vi "Stanford Research PS300 Series Configuration Display.vi"() -> ()   [LabVIEW 2013]
doc: "This VI first configures the instrument's setting (voltage/current) plus an associated value, commands the instrument to output the voltage, and finally returns a reading, showing the current display of the output source.\n\nNote: If Err 7 is generated by this VI Check to make sure that the High Vlotage Switch on the Instrument's Front Panel is turned ON, if it is OFF the high voltage will remain off and the instrument generates an execution error."
uses:
  Stanford Research PS300 Series.lvlib
panel:
  out "Display Reading":dbl=-49.0 format="%^.4e"
  in  "Voltage Setting (50.00)":dbl=50.0 format="%^.2e"
  in  "High Limit (1.00E+3)":dbl=1000.0 format="%^.2e"
  in  "Source Setting (T:Voltage)":bool=TRUE
  in  "error in (no error)":errorcluster {"code" format="%.0x"}
  out "VISA resource name out":refnum<visa-resource-name>
  in  "VISA resource name":refnum<visa-resource-name>
  # "(c) 2005-2015 National Instruments.  ALL RIGHTS RESERVED."
  # "Voltage\nCurrent"
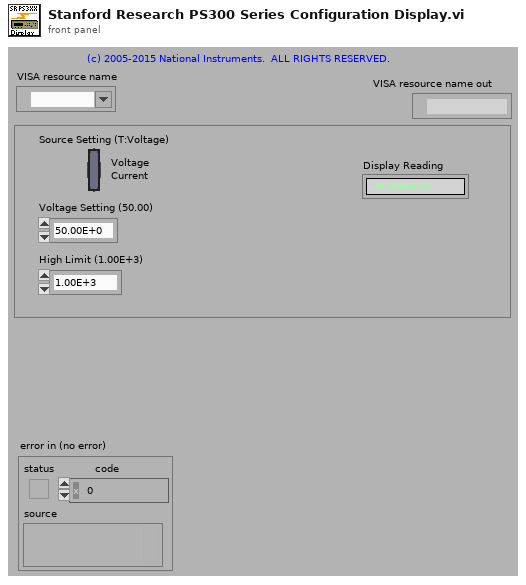
[diagram p1: front panel]
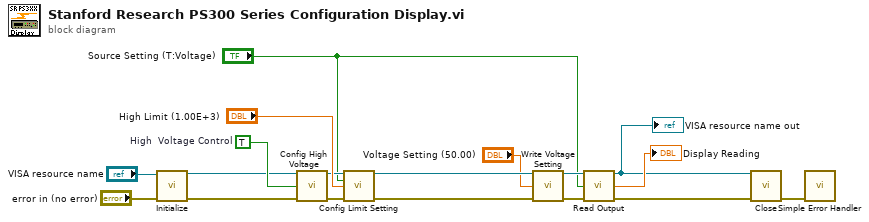
[diagram p0: block diagram]
diagram:
  w9 = TRUE  # High  Voltage Control
  n1 = call "Initialize.vi"("VISA resource name"="VISA resource name", "error in (no error)"="error in (no error)") -> ("VISA resource name out"=w7:refnum<visa-resource-name>, "error out"=w6:errorcluster)  [unwired: 12 in]
  n2 = call "Config High Voltage.vi"("VISA resource name"=w7, "High  Voltage Control (T:On)"=w9, "error in (no error)"=w6) -> ("VISA resource name out"=w11:refnum<visa-resource-name>, "error out"=w10:errorcluster)  [unwired: 11 in]
  n3 = call "Config Limit Setting.vi"("VISA resource name"=w11, "Source Setting (T:Voltage)"="Source Setting (T:Voltage)", "High Limit (1.00E+3)"="High Limit (1.00E+3)", "error in (no error)"=w10) -> ("VISA resource name out"=w18:refnum<visa-resource-name>, "error out"=w15:errorcluster)  [unwired: 10 in]
  n4 = call "Write Voltage Setting.vi"("VISA resource name"=w18, "Voltage Setting (100.00)"="Voltage Setting (50.00)", "error in (no error)"=w15) -> ("VISA resource name out"=w17:refnum<visa-resource-name>, "error out"=w16:errorcluster)  [unwired: 11 in]
  n5 = call "Read Output.vi"("VISA resource name"=w17, "Reading Source (T:Voltage)"="Source Setting (T:Voltage)", "error in (no error)"=w16) -> ("VISA resource name out"=w2:refnum<visa-resource-name>, "Display Reading"=→"Display Reading":dbl, "error out"=w3:errorcluster)  [unwired: 10 in]
  "VISA resource name out" <- w2
  n6 = call "Close.vi"("VISA resource name"=w2, "error in (no error)"=w3) -> ("error out"=w1:errorcluster)  [unwired: 13 in]
  n7 = call "Simple Error Handler.vi"("error in (no error)"=w1) -> ()  [unwired: 4 in, 5 out]
